vi "WW_Course_Spin_Parameter.vi"(0 "路径":path) -> (2 "PrjFinalSpinTime":T2, 3 "SpeedTime":T1, 4 "EXCEL读取":string[][](array[string]))   [LabVIEW 2011]
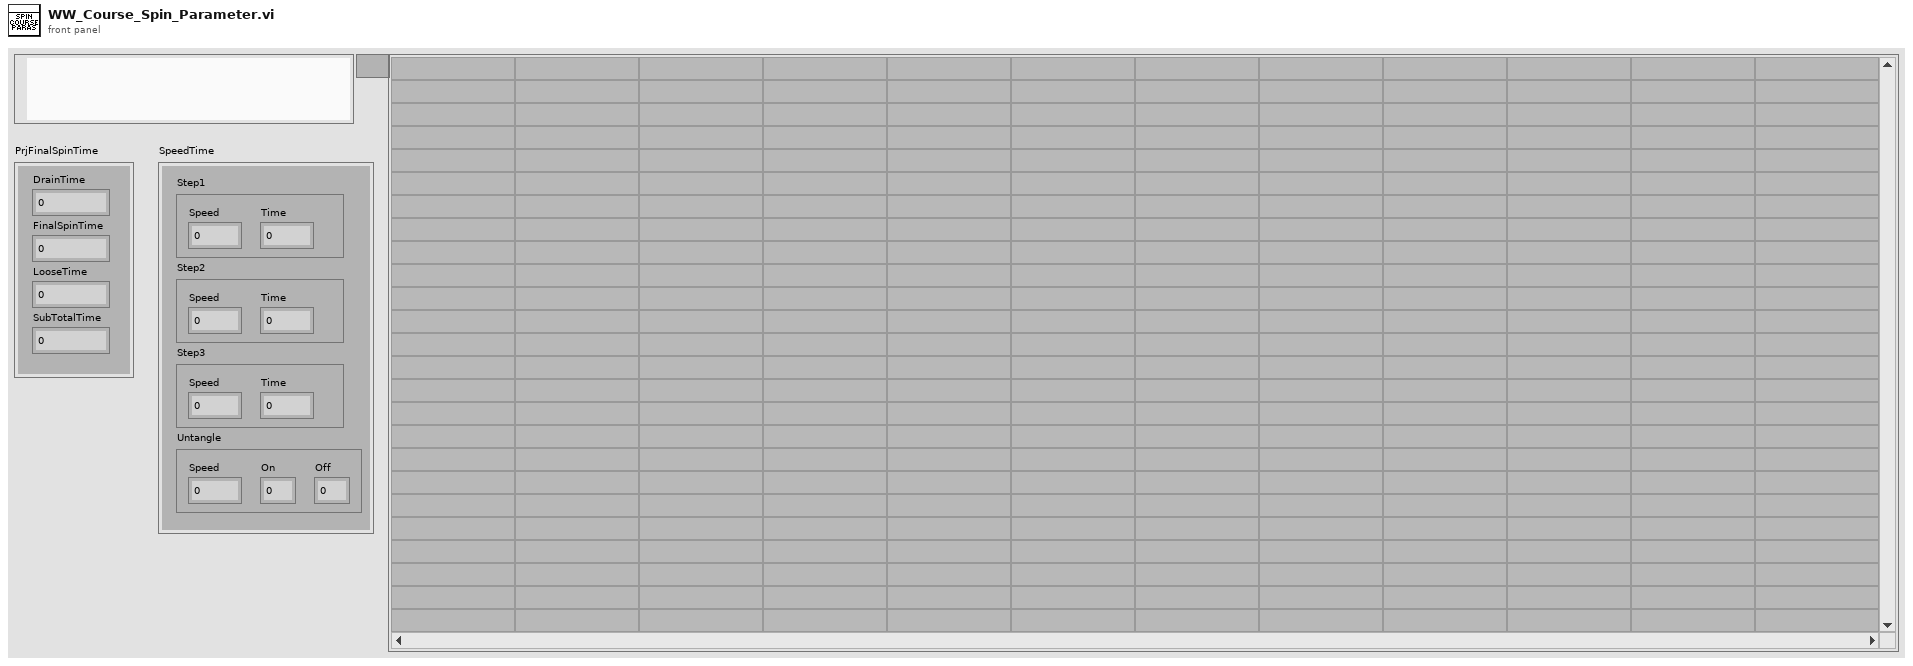
[diagram p1: front panel]
types:
  T1 = cluster{"Step1":cluster{"Speed":u32, "Time":u32}, "Step2":cluster{"Speed":u32, "Time":u32}, "Step3":cluster{"Speed":u32, "Time":u32}, "Untangle":cluster{"Speed":u32, "On":u32, "Off":u32}}
  T2 = cluster{"DrainTime":u32, "FinalSpinTime":u32, "LooseTime":u32, "SubTotalTime":u32}
  T3 = enum8{"NULL", "Course", "eCotton", "Synthetics", "Wool", "Spin", "RinseSpin", "EcoDrumClean", "DarkGarment", "OutDoorCare", "BabyCare", "Delicates", "Bedding", "SuperEcoWash", "SuperSpeed"}
  T4 = cluster{"Step1":cluster{"Speed":i32, "Time":i32}, "Step2":cluster{"Speed":i32, "Time":i32}, "Step3":cluster{"Speed":i32, "Time":i32}, "Untangle":cluster{"Speed":i32, "On":i32, "Off":i32}}
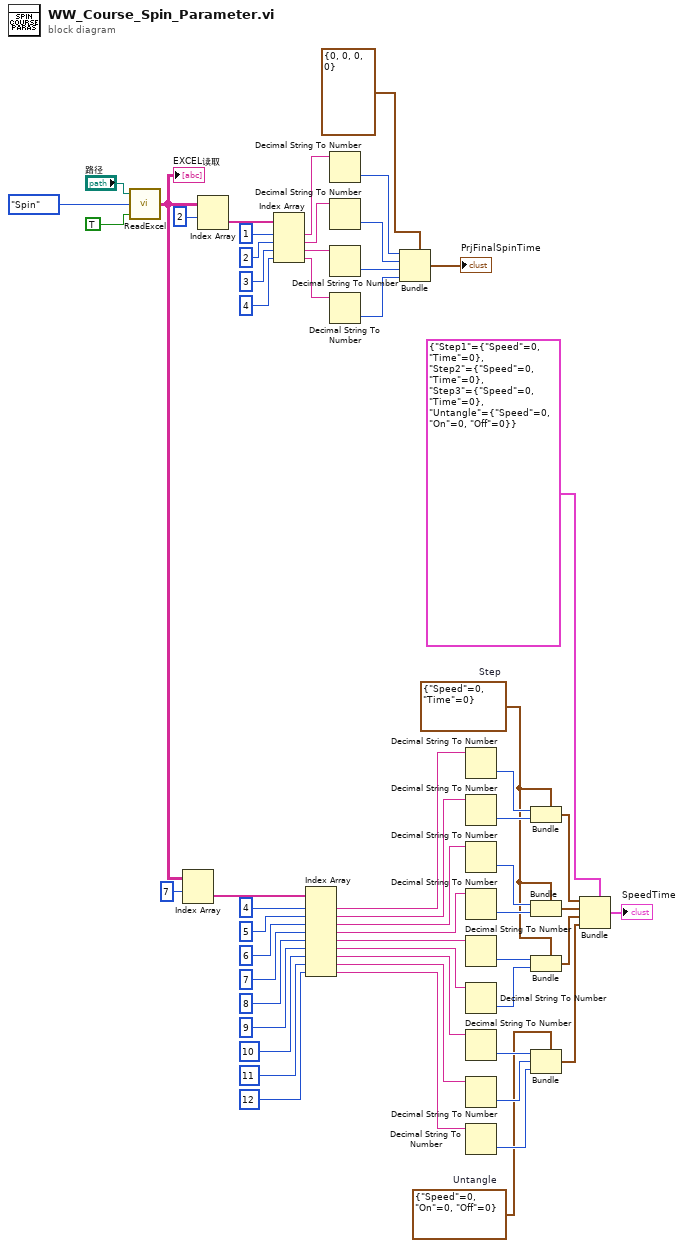
[diagram p0: block diagram]
diagram:
  w7 = cluster{"Speed":i32, "On":i32, "Off":i32} {"Speed"=0, "On"=0, "Off"=0}  # Untangle
  w8 = cluster{"Speed":i32, "Time":i32} {"Speed"=0, "Time"=0}  # Step
  n1 = call "ReadExcel.vi"("读出文本"=TRUE, "导出sheet位号"=T3."Spin" ("enumCourse"), "路径"="路径") -> ("EXCEL读取"=w9:string[][])
  "EXCEL读取" <- w9
  n2 = Index Array(array=w9, index (row)=7 ("索引 (行)")) -> (element=w10:string[])  [unwired: 1 in]
  n3 = Index Array(array=w9, index (row)=2 ("索引 (行)")) -> (element=w54:string[])  [unwired: 1 in]
  n4 = Index Array(array=w54, index #1=1 ("索引"), index #2=2 ("索引"), index #3=3 ("索引"), index #4=4 ("索引")) -> (element #1=w49:string, element #2=w46:string, element #3=w45:string, element #4=w44:string)
  n5 = Index Array(array=w10, index #1=4 ("索引"), index #2=5 ("索引"), index #3=6 ("索引"), index #4=7 ("索引"), index #5=8 ("索引"), index #6=9 ("索引"), index #7=10 ("索引"), index #8=11 ("索引"), index #9=12 ("索引")) -> (element #1=w13:string, element #2=w14:string, element #3=w19:string, element #4=w20:string, element #5=w25:string, element #6=w26:string, element #7=w32:string, element #8=w33:string, element #9=w34:string)
  n6 = Decimal String To Number(string=w49) -> (number=w47:i32)  [unwired: 2 in, 1 out]
  n7 = Decimal String To Number(string=w46) -> (number=w43:i32)  [unwired: 2 in, 1 out]
  n8 = Decimal String To Number(string=w45) -> (number=w42:i32)  [unwired: 2 in, 1 out]
  n9 = Decimal String To Number(string=w44) -> (number=w41:i32)  [unwired: 2 in, 1 out]
  n10 = Bundle(cluster=cluster{i32, i32, i32, i32} {0, 0, 0, 0} ("输入簇"), w47, w43, w42, w41) -> (→"PrjFinalSpinTime":cluster{i32, i32, i32, i32})
  n11 = Decimal String To Number(string=w13) -> (number=w15:i32)  [unwired: 2 in, 1 out]
  n12 = Decimal String To Number(string=w14) -> (number=w16:i32)  [unwired: 2 in, 1 out]
  n13 = Decimal String To Number(string=w19) -> (number=w21:i32)  [unwired: 2 in, 1 out]
  n14 = Decimal String To Number(string=w20) -> (number=w22:i32)  [unwired: 2 in, 1 out]
  n15 = Decimal String To Number(string=w25) -> (number=w28:i32)  [unwired: 2 in, 1 out]
  n16 = Decimal String To Number(string=w26) -> (number=w27:i32)  [unwired: 2 in, 1 out]
  n17 = Decimal String To Number(string=w32) -> (number=w35:i32)  [unwired: 2 in, 1 out]
  n18 = Decimal String To Number(string=w33) -> (number=w36:i32)  [unwired: 2 in, 1 out]
  n19 = Decimal String To Number(string=w34) -> (number=w37:i32)  [unwired: 2 in, 1 out]
  n20 = Bundle(cluster=w8, "Speed"=w15, "Time"=w16) -> (w6:cluster{"Speed":i32, "Time":i32})
  n21 = Bundle(cluster=w8, "Speed"=w21, "Time"=w22) -> (w5:cluster{"Speed":i32, "Time":i32})
  n22 = Bundle(cluster=w8, "Speed"=w28, "Time"=w27) -> (w4:cluster{"Speed":i32, "Time":i32})
  n23 = Bundle(cluster=w7, "Speed"=w35, "On"=w36, "Off"=w37) -> (w3:cluster{"Speed":i32, "On":i32, "Off":i32})
  n24 = Bundle(cluster=T4 {"Step1"={"Speed"=0, "Time"=0}, "Step2"={"Speed"=0, "Time"=0}, "Step3"={"Speed"=0, "Time"=0}, "Untangle"={"Speed"=0, "On"=0, "Off"=0}}, "Step1"=w6, "Step2"=w5, "Step3"=w4, "Untangle"=w3) -> (→"SpeedTime":T4)
